vi "Actor Core.vi"(8 "error in":errorcluster, 11 "Actor_Log in":refnum<class "Actor_EventStart.lvclass">) -> (0 "error out":errorcluster, 3 "Actor out":refnum<class "Actor.lvclass">)   [LabVIEW 2020, in "Library Core.lvlib" / "Actor_EventStart.lvlib" / "Actor_EventStart.lvclass"]
doc: "(<B>Filename</B>: Actor Framework.lvlib:Actor.lvclass:Actor Core.vi)\n\nReceives messages to the actor, reacts to them, and initiates any error handling that may shut the actor down.\n\nDescendant classes may override this VI to append parallel tasks for the actor to complete while it handles messages. Overrides use the Call Parent Method node."
uses:
  Actor_EventStart.lvclass
  C:/Program Files (x86)/National Instruments/LabVIEW 2020/vi.lib/ActorFramework/Actor/Actor.lvclass
  <vilib>/ActorFramework/Actor/Actor.lvclass
  Actor_EventStart.lvclass/Actor_EventStart.ctl
  Commun VI/TypeDef/Variable Printable.ctl
  Classe Event (Default)/Class Event (Default).lvclass
  <vilib>/ActorFramework/Actor/Actor.lvclass/Actor.ctl
  <vilib>/ActorFramework/Message Enqueuer/Message Enqueuer.lvclass/Message Enqueuer.ctl
  Actor_EventStart Messages/Message State/Message State.lvclass/Message State.ctl
  <vilib>/ActorFramework/Message Enqueuer/Init from Existing Queue.vi
  <vilib>/ActorFramework/Message Enqueuer/Enqueue.vi
  Actor_EventStart Messages/Message State/Message State.lvclass
  C:/Program Files (x86)/National Instruments/LabVIEW 2020/vi.lib/ActorFramework/Message/Message.lvclass
  <vilib>/ActorFramework/Message Priority Queue/Priority Enqueue.vi
  <vilib>/ActorFramework/Message Enqueuer/Message Enqueuer.lvclass
panel:
  out "Chaîne":string="Event Enabled"
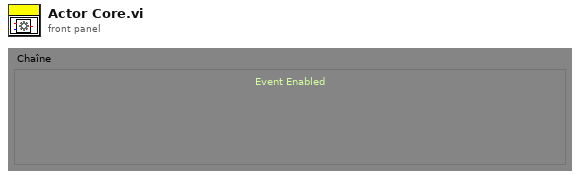
[diagram p1: front panel]
types:
  T1 = enum16{"Not Use", "Wait Event", "Test in progress", "Test Stopped"}
  T2 = typedef "Variable Printable.ctl" = string
  T3 = enum16{"Get Variable", "Get All Variables", "Set Variable", "Delete Variable", "Delete All Variable"}
  T4 = enum32{"Invalid", "Standard", "Closed", "Hidden", "Minimized", "Maximized"}
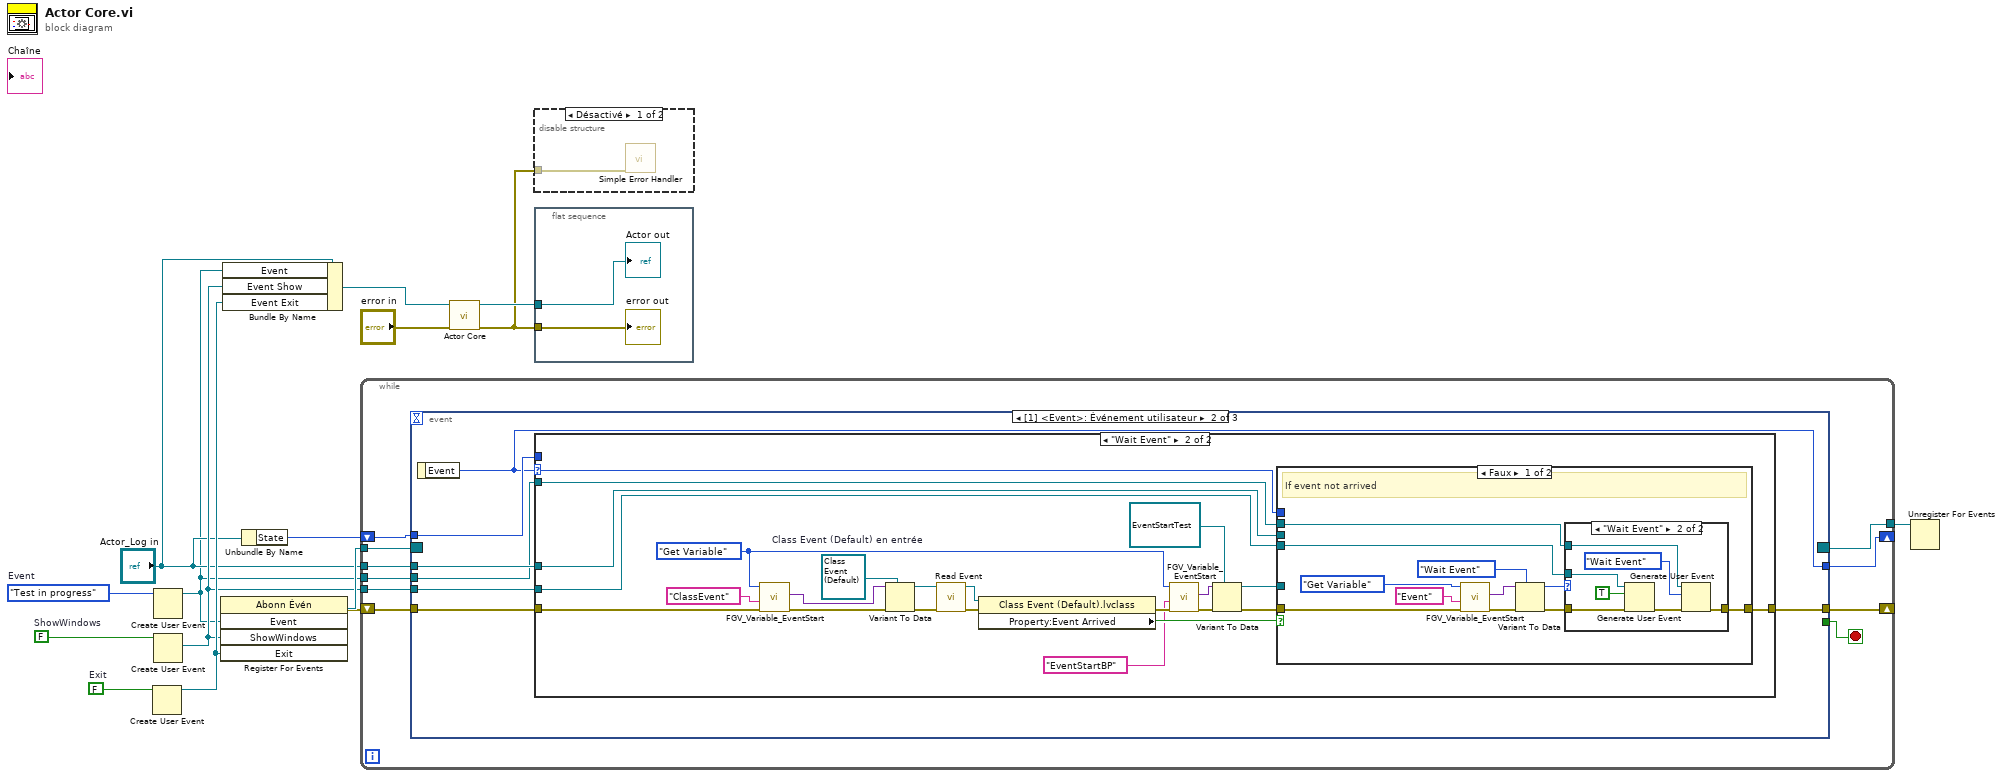
[diagram p0: block diagram]
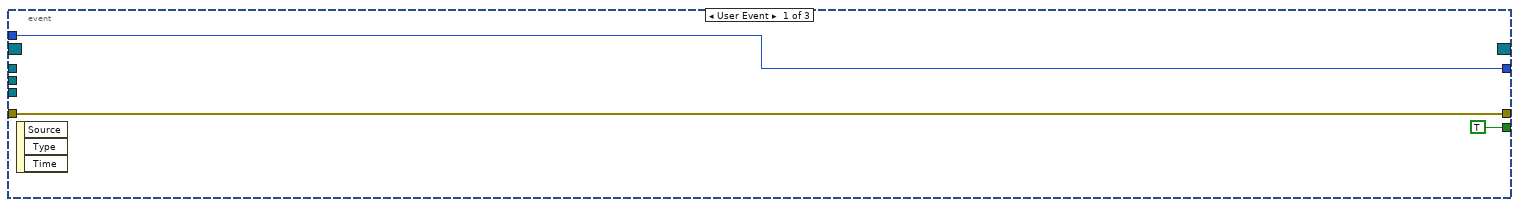
[diagram p3: hidden frame]
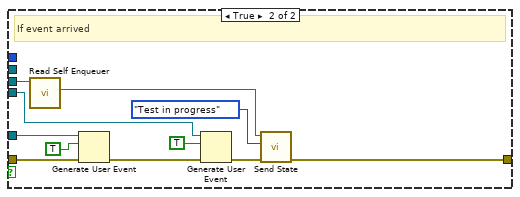
[diagram p6: hidden frame]
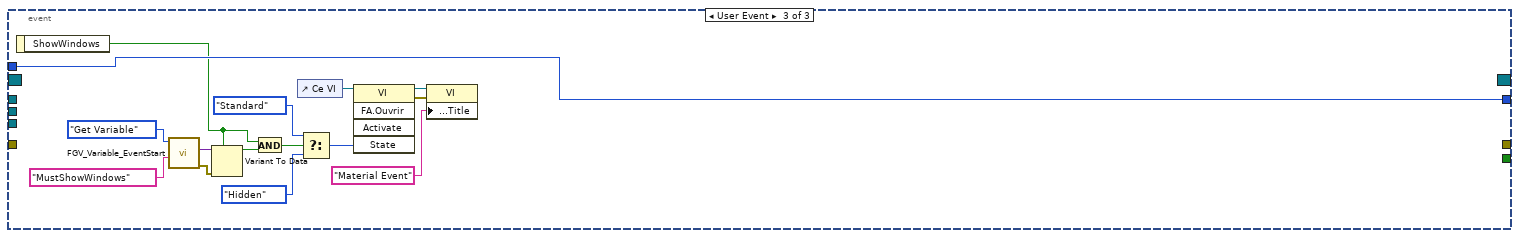
[diagram p7: hidden frame]
diagram:
  w5 = FALSE  # ShowWindows
  w7 = T1."Test in progress"  # Event
  w9 = FALSE  # Exit
  n1 = Create User Event(user event datatype=w9) -> (user event=w8:refnum<user-event>)  [unwired: 1 in, 1 out]
  n2 = Create User Event(user event datatype=w7) -> (user event=w1:refnum<user-event>)  [unwired: 1 in, 1 out]
  n3 = Create User Event(user event datatype=w5) -> (user event=w4:refnum<user-event>)  [unwired: 1 in, 1 out]
  n4 = register-events(w1, w4, w8) -> (reference out=w12:refnum<event-registration>, error out=w6:errorcluster)  [unwired: 2 in]
  n5 = Bundle By Name(cluster="Actor_Log in", "Event"=w1, "Event Show"=w4, "Event Exit"=w8) -> (w13:refnum<class "Actor_EventStart.lvclass">)
  n6 = Unbundle By Name("Actor_Log in") -> ("State"=w2:T1)
  n7 = while {
    tunnel: w12 -> [w25]
    tunnel: [w24] -> w11
    tunnel: "Actor_Log in" -> [w23]
    tunnel: w1 -> [w21]
    shift-right: [w19] -> _
    shift-left: w6 -> [w20]
    tunnel: w4 -> [w18]
    shift-right: [w16] -> _
    shift-left: w2 -> [w17]
    stop <- w22 stop-if-true
    n8 = event shown="[1] <Event>: Événement utilisateur" {
      selector: w25 -> [_ _ _]
      dyn-events: [_ _ _] -> w24
      timeout: _ -> [_ _ _]
      tunnel: w23 -> [_ w35 _]
      tunnel: [TRUE _ _] -> w22
      tunnel: w21 -> [_ w32 _]
      tunnel: w20 -> [w27 w34 _]
      tunnel: [w27 w33 _] -> w19
      tunnel: w18 -> [_ w31 _]
      tunnel: w17 -> [w26 w30 w96]
      tunnel: [w26 w29 w96] -> w16
      event User Event {
        n9 = event-data() -> ()  [unwired: 1 in, 3 out]
      }
      event User Event {
        n10 = event-data() -> ("Event"=w29:T1)  [unwired: 1 in]
        n11 = case shown="\"Wait Event\"" w29 {
          selector: w29 -> [_ w54]
          tunnel: w35 -> [_ w52]
          tunnel: w34 -> [w36 w47]
          tunnel: [w36 w56] -> w33
          tunnel: w32 -> [_ w55]
          tunnel: w31 -> [_ w53]
          tunnel: w30 -> [_ _]
          frame "Not Use", Default {
          }
          frame "Wait Event" {
            w49 = refnum<class "Class Event (Default).lvclass"> refnum  # Class Event (Default) en entrée
            w41 = T3."Get Variable" ("Function")
            n12 = call "FGV_Variable_EventStart.vi"("error in (no error)"=w47, "Variable"=T2 "ClassEvent", "Function"=w41) -> ("error out"=w50:errorcluster, "Data Out"=w45:variant)  [unwired: 6 in, 1 out]
            n13 = Variant To Data(error in=w50, type=w49, Variant=w45) -> (data=w48:refnum<class "Class Event (Default).lvclass">, error out=w46:errorcluster)
            n14 = call-dynamic "Read Event.vi"("error in (no error)"=w46, "Class Event (Default) en entrée"=w48) -> ("error out"=w58:errorcluster, "Class Event (Default) en sortie"=w59:refnum<class "Class Event (Default).lvclass">)  [unwired: 8 in]
            n15 = property class="Class Event (Default).lvclass"(reference=w59, error in=w58) -> (error out=w44:errorcluster, "Property:Event Arrived"=w57:bool)  [unwired: 1 out]
            n16 = call "FGV_Variable_EventStart.vi"("error in (no error)"=w44, "Variable"=T2 "EventStartBP", "Function"=w41) -> ("error out"=w43:errorcluster, "Data Out"=w40:variant)  [unwired: 6 in, 1 out]
            n17 = Variant To Data(error in=w43, type=refnum<user-event> refnum ("Parameter.Event Start BP"), Variant=w40) -> (data=w38:refnum<user-event>, error out=w42:errorcluster)
            n18 = case shown="Faux" w57 {
              tunnel: w38 -> [_ w89]
              tunnel: w42 -> [w60 w87]
              tunnel: [w70 w81] -> w56
              tunnel: w55 -> [w69 _]
              tunnel: w54 -> [_ _]
              tunnel: w53 -> [w61 w84]
              tunnel: w52 -> [_ w83]
              frame False {
                # "If event not arrived"
                n19 = call "FGV_Variable_EventStart.vi"("error in (no error)"=w60, "Variable"=T2 "Event", "Function"=T3."Get Variable") -> ("error out"=w67:errorcluster, "Data Out"=w68:variant)  [unwired: 6 in, 1 out]
                n20 = Variant To Data(error in=w67, type=T1."Wait Event" ("données d'événement"), Variant=w68) -> (data=w62:T1, error out=w63:errorcluster)
                n21 = case shown="\"Wait Event\"" w62 {
                  tunnel: [w71 w78] -> w70
                  tunnel: w69 -> [_ w77]
                  tunnel: w63 -> [w71 w73]
                  tunnel: w61 -> [_ w75]
                  frame "Not Use", Default {
                  }
                  frame "Wait Event" {
                    n22 = Generate User Event(user event=w75, event data cluster=TRUE ("données d'événement"), error in=w73) -> (error out=w72:errorcluster)  [unwired: 1 in, 1 out]
                    n23 = Generate User Event(user event=w77, event data cluster=T1."Wait Event" ("données d'événement"), error in=w72) -> (error out=w78:errorcluster)  [unwired: 1 in, 1 out]
                  }
                }
              }
              frame True {
                # "If event arrived"
                n24 = call <vilib>:"Read Self Enqueuer.vi"("Actor"=w83) -> ("Self Enqueuer"=w80:refnum<class "Message Enqueuer.lvclass">)  [unwired: 10 in]
                n25 = Generate User Event(user event=w89, event data cluster=TRUE ("données d'événement"), error in=w87) -> (error out=w85:errorcluster)  [unwired: 1 in, 1 out]
                n26 = Generate User Event(user event=w84, event data cluster=TRUE ("données d'événement"), error in=w85) -> (error out=w82:errorcluster)  [unwired: 1 in, 1 out]
                n27 = call "Send State.vi"("error in (no error)"=w82, "State"=T1."Test in progress", "Message Enqueuer"=w80) -> ("error out"=w81:errorcluster)  [unwired: 7 in, 1 out]
              }
            }
          }
        }
      }
      event User Event {
        n28 = event-data() -> ("ShowWindows"=w91:bool)  [unwired: 1 in]
        n29 = call "FGV_Variable_EventStart.vi"("Variable"=T2 "MustShowWindows", "Function"=T3."Get Variable") -> ("error out"=w93:errorcluster, "Data Out"=w92:variant)  [unwired: 7 in, 1 out]
        n30 = Variant To Data(error in=w93, type=w91, Variant=w92) -> (data=w90:bool)  [unwired: 1 out]
        n31 = And(x=w91, y=w90) -> (x .and. y?=w97:bool)
        n32 = control-ref of="Ce VI"() -> (w104:refnum<vi>)
        n33 = Select(t=T4."Standard" ("État"), s=w97, f=T4."Hidden" ("État")) -> (s? t:f=w101:T4)
        n34 = invoke class="VI" method="FA.Ouvrir"(reference=w104, "State"=w101) -> (reference out=w102:refnum<vi>, error out=w103:errorcluster)  [unwired: 3 in, 3 out]
        n35 = property class="VI"(reference=w102, error in=w103, "Front Panel.Title"="Material Event" ("Fenêtre face-avant:Titre")) -> ()  [unwired: 2 out]
      }
    }
  }
  n36 = call-parent "Actor Core.vi"("error in"="error in", "Actor in"=w13) -> ("error out"=w10:errorcluster, "Actor out"=w15:refnum<class "Actor.lvclass">)  [unwired: 8 in]
  n37 = disable-structure shown="Désactivé" {
    disable-tunnel: w10 -> [w105 _]
    frame Disabled {
      n38 = call <vilib>:"Simple Error Handler.vi"("error in (no error)"=w105) -> ()  [unwired: 4 in, 5 out]
    }
    frame Enabled {
    }
  }
  n39 = flat-sequence {
    tunnel: w10 -> [w107]
    tunnel: w15 -> [w106]
    frame #0 {
      "error out" <- w107
      "Actor out" <- w106
    }
  }
  n40 = Unregister For Events(event registration refnum=w11) -> ()  [unwired: 1 in, 1 out]
